vi "Auto Loop 1.vi"(2 "Auto State":u8, 3 "Call Context":T4) -> (0 "Loop 1 Data":T1, 1 "SubState 1":T2)   [LabVIEW 2014]
uses:
  <vilib>/Rock Robotics/WPI/DriverStation/WPI_DriverStationDerivedRobotMode.ctl
  typedefs/state machine/subStates.ctl
  typedefs/loop datatypes/Loop 1 Datatype.ctl
  typedefs/lift/lift command.ctl
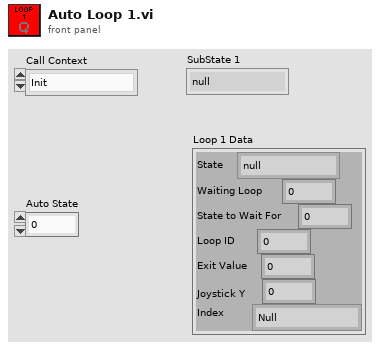
[diagram p1: front panel]
types:
  T1 = typedef "Loop 1 Datatype.ctl" = cluster{"State":T2, "Waiting Loop":i32, "State to Wait For":i32, "Loop ID":i32, "Exit Value":i32, "Joystick Y":dbl, "Index":T3}
  T2 = typedef "subStates.ctl" = enum16{"null", "wait", "driver control", "auto", "manual override", "hold position", "rotate", "test", "end"}
  T3 = typedef "lift command.ctl" = enum16{"Null", "Index Up", "Index Down", "Go To Home", "Cap 4 Stack", "Container Index Up", "Container Index Down", "Autonomous"}
  T4 = typedef "WPI_DriverStationDerivedRobotMode.ctl" = enum16{"Init", "Execute", "Stop"}
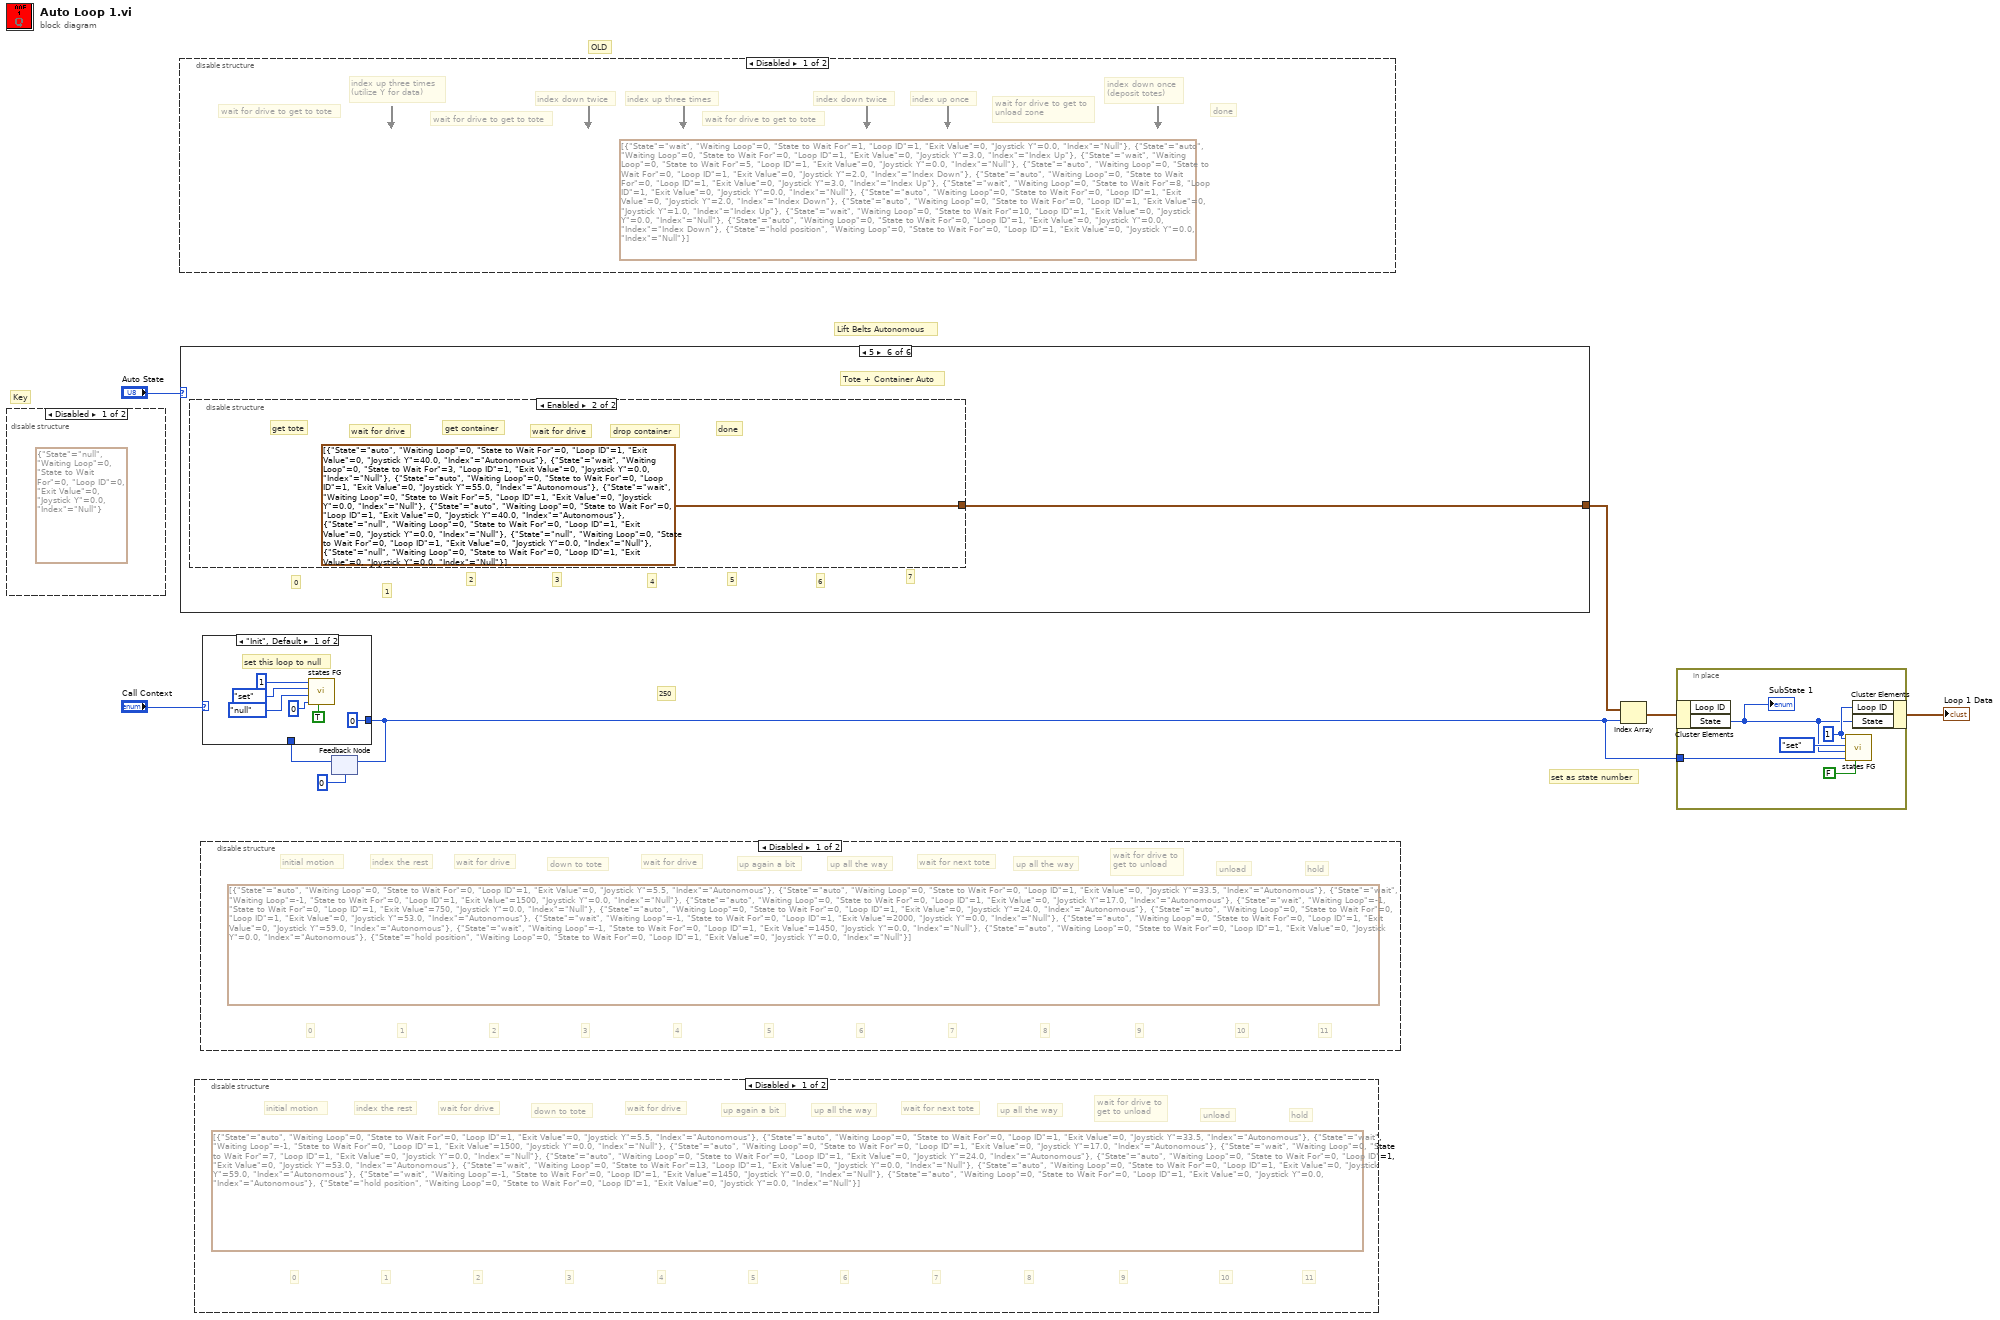
[diagram p0: block diagram]
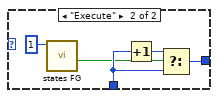
[diagram p6: hidden frame]
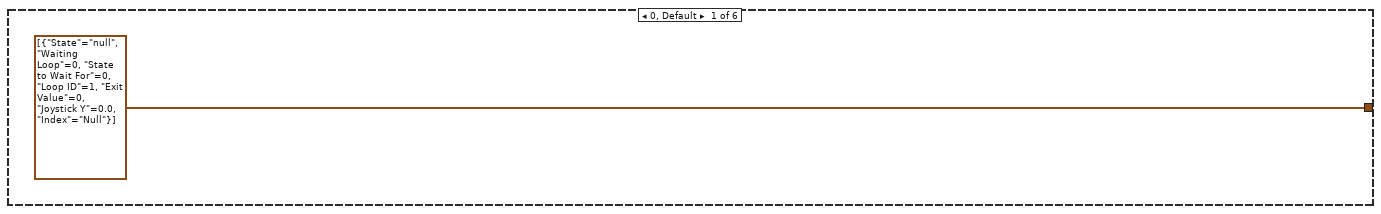
[diagram p7: hidden frame]
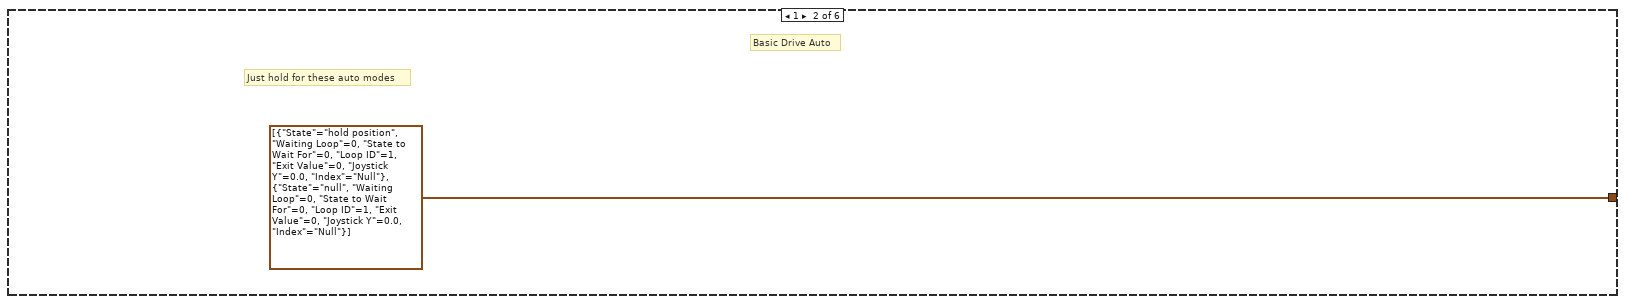
[diagram p8: hidden frame]
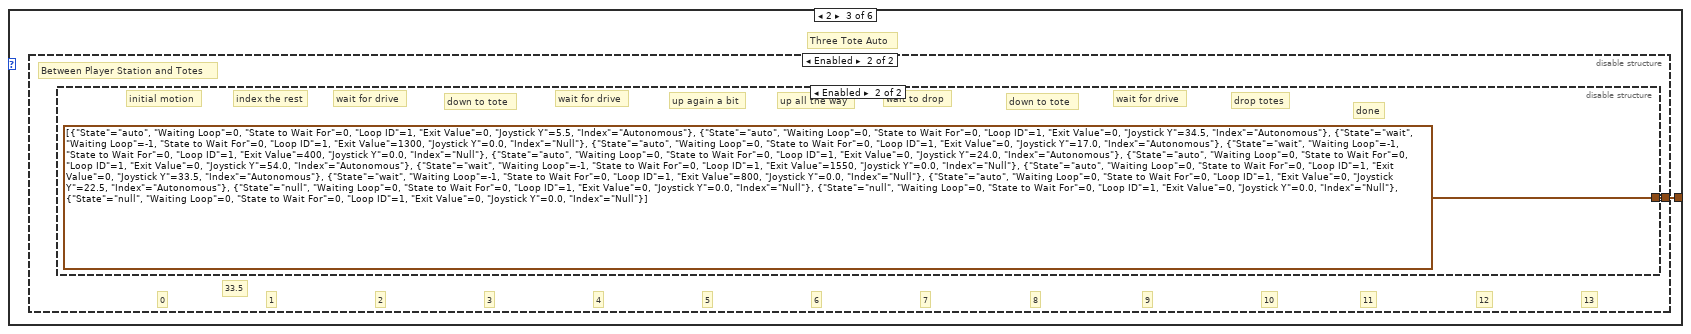
[diagram p9: hidden frame]
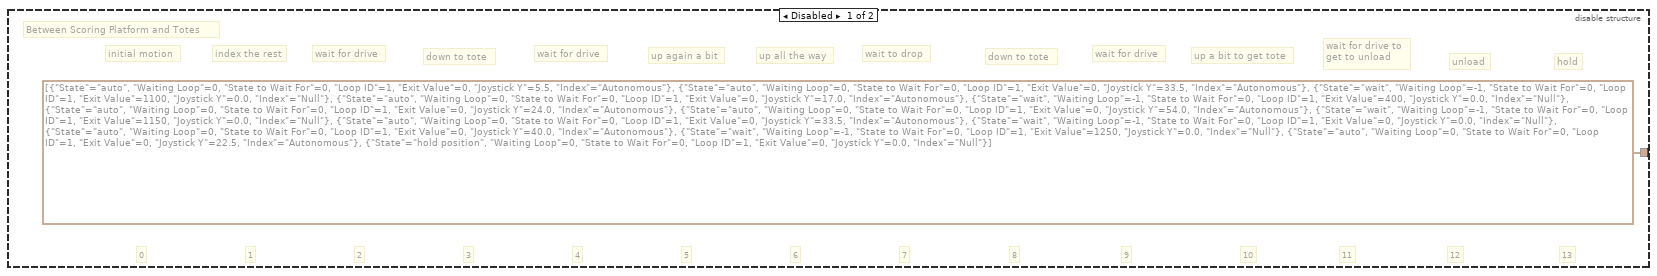
[diagram p10: hidden frame]
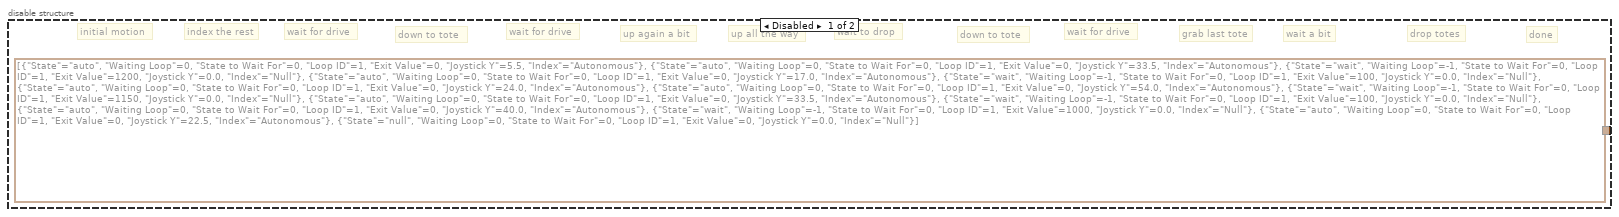
[diagram p11: hidden frame]
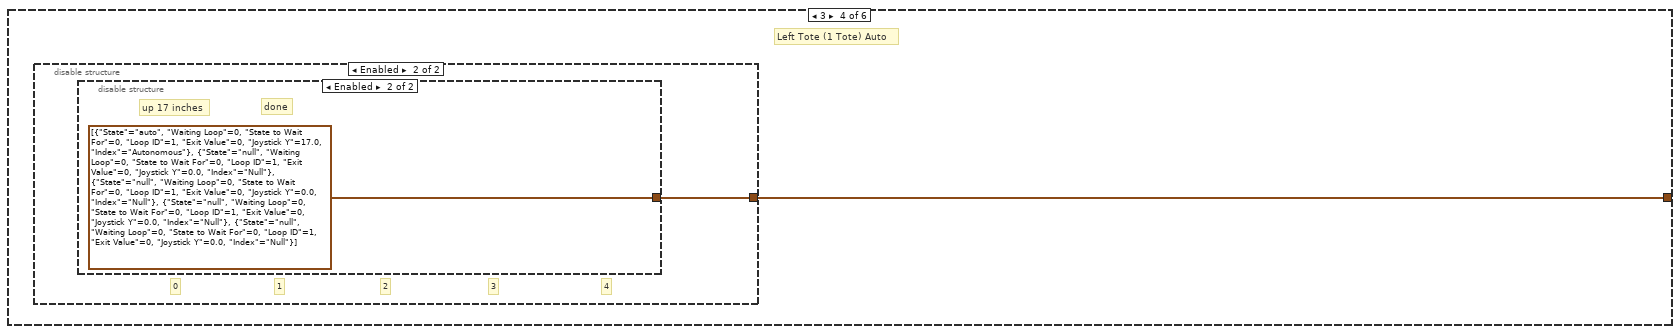
[diagram p12: hidden frame]
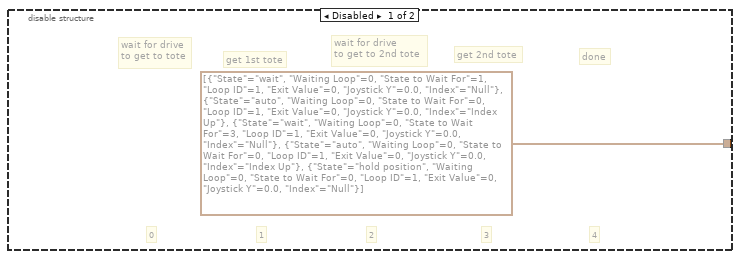
[diagram p13: hidden frame]
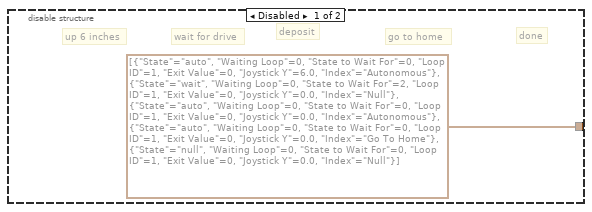
[diagram p14: hidden frame]
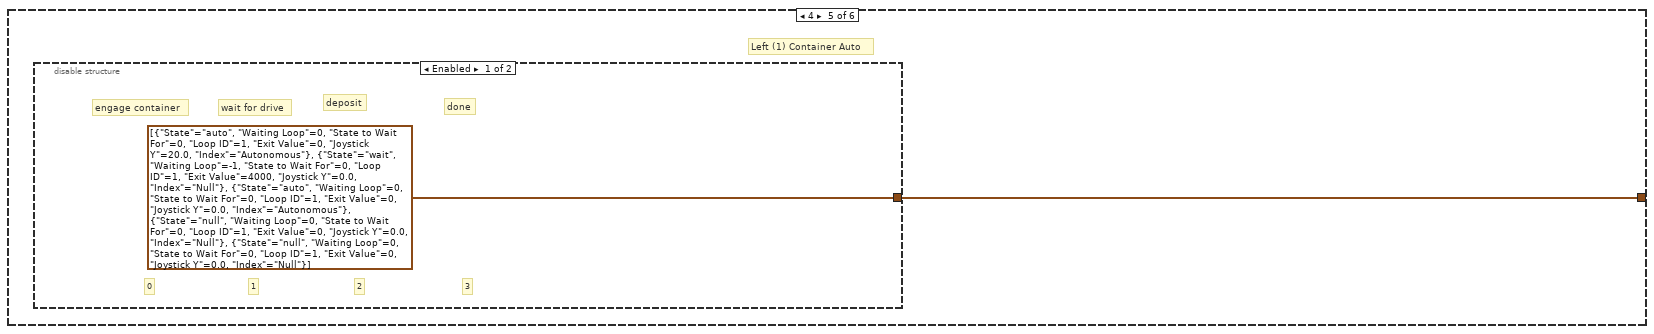
[diagram p15: hidden frame]
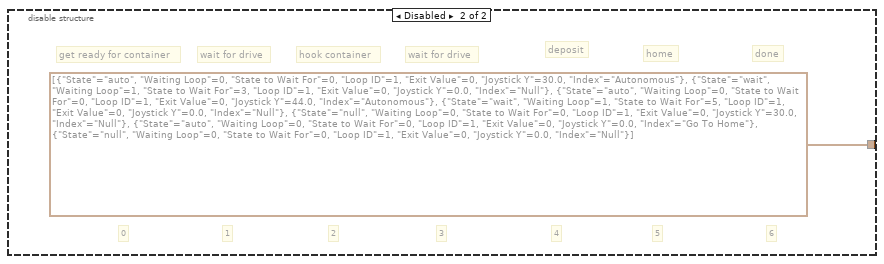
[diagram p16: hidden frame]
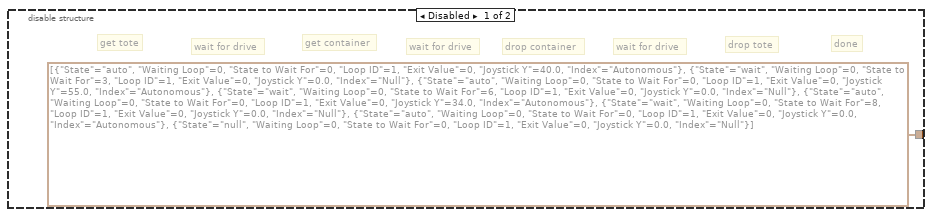
[diagram p17: hidden frame]
diagram:
  # "250"
  # "OLD"
  # "set as state number"
  # "Key"
  # "Lift Belts Autonomous"
  n1 = disable-structure shown="Disabled" {
    frame Disabled {
      (unwired) T1 {"State"=enum."null", "Waiting Loop"=0, "State to Wait For"=0, "Loop ID"=0, "Exit Value"=0, "Joystick Y"=0.0, "Index"=enum."Null"} ("Loop 1 Data")
    }
    frame Enabled {
    }
  }
  n2 = disable-structure shown="Disabled" {
    frame Disabled {
      (unwired) T1[] [{"State"=enum."wait", "Waiting Loop"=0, "State to Wait For"=1, "Loop ID"=1, "Exit Value"=0, "Joystick Y"=0.0, "Index"=enum."Null"}, {"State"=enum."auto", "Waiting Loop"=0, "State to Wait For"=0, "Loop ID"=1, "Exit Value"=0, "Joystick Y"=3.0, "Index"=enum."Index Up"}, {"State"=enum."wait", "Waiting Loop"=0, "State to Wait For"=5, "Loop ID"=1, "Exit Value"=0, "Joystick Y"=0.0, "Index"=enum."Null"}, {"State"=enum."auto", "Waiting Loop"=0, "State to Wait For"=0, "Loop ID"=1, "Exit Value"=0, "Joystick Y"=2.0, "Index"=enum."Index Down"}, {"State"=enum."auto", "Waiting Loop"=0, "State to Wait For"=0, "Loop ID"=1, "Exit Value"=0, "Joystick Y"=3.0, "Index"=enum."Index Up"}, {"State"=enum."wait", "Waiting Loop"=0, "State to Wait For"=8, "Loop ID"=1, "Exit Value"=0, "Joystick Y"=0.0, "Index"=enum."Null"}, {"State"=enum."auto", "Waiting Loop"=0, "State to Wait For"=0, "Loop ID"=1, "Exit Value"=0, "Joystick Y"=2.0, "Index"=enum."Index Down"}, {"State"=enum."auto", "Waiting Loop"=0, "State to Wait For"=0, "Loop ID"=1, "Exit Value"=0, "Joystick Y"=1.0, "Index"=enum."Index Up"}, {"State"=enum."wait", "Waiting Loop"=0, "State to Wait For"=10, "Loop ID"=1, "Exit Value"=0, "Joystick Y"=0.0, "Index"=enum."Null"}, {"State"=enum."auto", "Waiting Loop"=0, "State to Wait For"=0, "Loop ID"=1, "Exit Value"=0, "Joystick Y"=0.0, "Index"=enum."Index Down"}, {"State"=enum."hold position", "Waiting Loop"=0, "State to Wait For"=0, "Loop ID"=1, "Exit Value"=0, "Joystick Y"=0.0, "Index"=enum."Null"}]
      # "done"
      # "index down once\n(deposit totes)"
      # "wait for drive to get to\nunload zone"
      # "index up once"
      # "index down twice"
      # "wait for drive to get to tote"
      # "index up three times"
      # "index down twice"
      # "wait for drive to get to tote"
      # "index up three times \n(utilize Y for data)"
      # "wait for drive to get to tote"
    }
    frame Enabled {
    }
  }
  n3 = case shown="5" "Auto State" {
    tunnel: [T1[] [{"State"=enum."null", "Waiting Loop"=0, "State to Wait For"=0, "Loop ID"=1, "Exit Value"=0, "Joystick Y"=0.0, "Index"=enum."Null"}] T1[] [{"State"=enum."hold position", "Waiting Loop"=0, "State to Wait For"=0, "Loop ID"=1, "Exit Value"=0, "Joystick Y"=0.0, "Index"=enum."Null"}, {"State"=enum."null", "Waiting Loop"=0, "State to Wait For"=0, "Loop ID"=1, "Exit Value"=0, "Joystick Y"=0.0, "Index"=enum."Null"}] w11 w16 w21 w24] -> w4
    frame 0, Default {
    }
    frame 1 {
      # "Basic Drive Auto"
      # "Just hold for these auto modes"
    }
    frame 2 {
      # "Three Tote Auto"
      n4 = disable-structure shown="Enabled" {
        disable-tunnel: [T1[] [{"State"=enum."auto", "Waiting Loop"=0, "State to Wait For"=0, "Loop ID"=1, "Exit Value"=0, "Joystick Y"=5.5, "Index"=enum."Autonomous"}, {"State"=enum."auto", "Waiting Loop"=0, "State to Wait For"=0, "Loop ID"=1, "Exit Value"=0, "Joystick Y"=33.5, "Index"=enum."Autonomous"}, {"State"=enum."wait", "Waiting Loop"=-1, "State to Wait For"=0, "Loop ID"=1, "Exit Value"=1100, "Joystick Y"=0.0, "Index"=enum."Null"}, {"State"=enum."auto", "Waiting Loop"=0, "State to Wait For"=0, "Loop ID"=1, "Exit Value"=0, "Joystick Y"=17.0, "Index"=enum."Autonomous"}, {"State"=enum."wait", "Waiting Loop"=-1, "State to Wait For"=0, "Loop ID"=1, "Exit Value"=400, "Joystick Y"=0.0, "Index"=enum."Null"}, {"State"=enum."auto", "Waiting Loop"=0, "State to Wait For"=0, "Loop ID"=1, "Exit Value"=0, "Joystick Y"=24.0, "Index"=enum."Autonomous"}, {"State"=enum."auto", "Waiting Loop"=0, "State to Wait For"=0, "Loop ID"=1, "Exit Value"=0, "Joystick Y"=54.0, "Index"=enum."Autonomous"}, {"State"=enum."wait", "Waiting Loop"=-1, "State to Wait For"=0, "Loop ID"=1, "Exit Value"=1150, "Joystick Y"=0.0, "Index"=enum."Null"}, {"State"=enum."auto", "Waiting Loop"=0, "State to Wait For"=0, "Loop ID"=1, "Exit Value"=0, "Joystick Y"=33.5, "Index"=enum."Autonomous"}, {"State"=enum."wait", "Waiting Loop"=-1, "State to Wait For"=0, "Loop ID"=1, "Exit Value"=0, "Joystick Y"=0.0, "Index"=enum."Null"}, {"State"=enum."auto", "Waiting Loop"=0, "State to Wait For"=0, "Loop ID"=1, "Exit Value"=0, "Joystick Y"=40.0, "Index"=enum."Autonomous"}, {"State"=enum."wait", "Waiting Loop"=-1, "State to Wait For"=0, "Loop ID"=1, "Exit Value"=1250, "Joystick Y"=0.0, "Index"=enum."Null"}, {"State"=enum."auto", "Waiting Loop"=0, "State to Wait For"=0, "Loop ID"=1, "Exit Value"=0, "Joystick Y"=22.5, "Index"=enum."Autonomous"}, {"State"=enum."hold position", "Waiting Loop"=0, "State to Wait For"=0, "Loop ID"=1, "Exit Value"=0, "Joystick Y"=0.0, "Index"=enum."Null"}] w13] -> w11
        frame Disabled {
          # "Between Scoring Platform and Totes"
          # "13"
          # "12"
          # "wait for drive"
          # "down to tote"
          # "11"
          # "hold"
          # "10"
          # "9"
          # "8"
          # "wait for drive to\nget to unload"
          # "up a bit to get tote"
          # "wait to drop"
          # "unload"
          # "wait for drive"
          # "up all the way"
          # "up again a bit"
          # "down to tote"
          # "wait for drive"
          # "index the rest"
          # "initial motion"
          # "7"
          # "6"
          # "5"
          # "4"
          # "3"
          # "2"
          # "1"
          # "0"
        }
        frame Enabled {
          # "33.5"
          # "13"
          # "12"
          # "Between Player Station and Totes"
          # "11"
          # "10"
          # "9"
          # "8"
          # "7"
          # "6"
          # "5"
          # "4"
          # "3"
          # "2"
          # "1"
          # "0"
          n5 = disable-structure shown="Enabled" {
            disable-tunnel: [T1[] [{"State"=enum."auto", "Waiting Loop"=0, "State to Wait For"=0, "Loop ID"=1, "Exit Value"=0, "Joystick Y"=5.5, "Index"=enum."Autonomous"}, {"State"=enum."auto", "Waiting Loop"=0, "State to Wait For"=0, "Loop ID"=1, "Exit Value"=0, "Joystick Y"=33.5, "Index"=enum."Autonomous"}, {"State"=enum."wait", "Waiting Loop"=-1, "State to Wait For"=0, "Loop ID"=1, "Exit Value"=1200, "Joystick Y"=0.0, "Index"=enum."Null"}, {"State"=enum."auto", "Waiting Loop"=0, "State to Wait For"=0, "Loop ID"=1, "Exit Value"=0, "Joystick Y"=17.0, "Index"=enum."Autonomous"}, {"State"=enum."wait", "Waiting Loop"=-1, "State to Wait For"=0, "Loop ID"=1, "Exit Value"=100, "Joystick Y"=0.0, "Index"=enum."Null"}, {"State"=enum."auto", "Waiting Loop"=0, "State to Wait For"=0, "Loop ID"=1, "Exit Value"=0, "Joystick Y"=24.0, "Index"=enum."Autonomous"}, {"State"=enum."auto", "Waiting Loop"=0, "State to Wait For"=0, "Loop ID"=1, "Exit Value"=0, "Joystick Y"=54.0, "Index"=enum."Autonomous"}, {"State"=enum."wait", "Waiting Loop"=-1, "State to Wait For"=0, "Loop ID"=1, "Exit Value"=1150, "Joystick Y"=0.0, "Index"=enum."Null"}, {"State"=enum."auto", "Waiting Loop"=0, "State to Wait For"=0, "Loop ID"=1, "Exit Value"=0, "Joystick Y"=33.5, "Index"=enum."Autonomous"}, {"State"=enum."wait", "Waiting Loop"=-1, "State to Wait For"=0, "Loop ID"=1, "Exit Value"=100, "Joystick Y"=0.0, "Index"=enum."Null"}, {"State"=enum."auto", "Waiting Loop"=0, "State to Wait For"=0, "Loop ID"=1, "Exit Value"=0, "Joystick Y"=40.0, "Index"=enum."Autonomous"}, {"State"=enum."wait", "Waiting Loop"=-1, "State to Wait For"=0, "Loop ID"=1, "Exit Value"=1000, "Joystick Y"=0.0, "Index"=enum."Null"}, {"State"=enum."auto", "Waiting Loop"=0, "State to Wait For"=0, "Loop ID"=1, "Exit Value"=0, "Joystick Y"=22.5, "Index"=enum."Autonomous"}, {"State"=enum."null", "Waiting Loop"=0, "State to Wait For"=0, "Loop ID"=1, "Exit Value"=0, "Joystick Y"=0.0, "Index"=enum."Null"}] T1[] [{"State"=enum."auto", "Waiting Loop"=0, "State to Wait For"=0, "Loop ID"=1, "Exit Value"=0, "Joystick Y"=5.5, "Index"=enum."Autonomous"}, {"State"=enum."auto", "Waiting Loop"=0, "State to Wait For"=0, "Loop ID"=1, "Exit Value"=0, "Joystick Y"=34.5, "Index"=enum."Autonomous"}, {"State"=enum."wait", "Waiting Loop"=-1, "State to Wait For"=0, "Loop ID"=1, "Exit Value"=1300, "Joystick Y"=0.0, "Index"=enum."Null"}, {"State"=enum."auto", "Waiting Loop"=0, "State to Wait For"=0, "Loop ID"=1, "Exit Value"=0, "Joystick Y"=17.0, "Index"=enum."Autonomous"}, {"State"=enum."wait", "Waiting Loop"=-1, "State to Wait For"=0, "Loop ID"=1, "Exit Value"=400, "Joystick Y"=0.0, "Index"=enum."Null"}, {"State"=enum."auto", "Waiting Loop"=0, "State to Wait For"=0, "Loop ID"=1, "Exit Value"=0, "Joystick Y"=24.0, "Index"=enum."Autonomous"}, {"State"=enum."auto", "Waiting Loop"=0, "State to Wait For"=0, "Loop ID"=1, "Exit Value"=0, "Joystick Y"=54.0, "Index"=enum."Autonomous"}, {"State"=enum."wait", "Waiting Loop"=-1, "State to Wait For"=0, "Loop ID"=1, "Exit Value"=1550, "Joystick Y"=0.0, "Index"=enum."Null"}, {"State"=enum."auto", "Waiting Loop"=0, "State to Wait For"=0, "Loop ID"=1, "Exit Value"=0, "Joystick Y"=33.5, "Index"=enum."Autonomous"}, {"State"=enum."wait", "Waiting Loop"=-1, "State to Wait For"=0, "Loop ID"=1, "Exit Value"=800, "Joystick Y"=0.0, "Index"=enum."Null"}, {"State"=enum."auto", "Waiting Loop"=0, "State to Wait For"=0, "Loop ID"=1, "Exit Value"=0, "Joystick Y"=22.5, "Index"=enum."Autonomous"}, {"State"=enum."null", "Waiting Loop"=0, "State to Wait For"=0, "Loop ID"=1, "Exit Value"=0, "Joystick Y"=0.0, "Index"=enum."Null"}, {"State"=enum."null", "Waiting Loop"=0, "State to Wait For"=0, "Loop ID"=1, "Exit Value"=0, "Joystick Y"=0.0, "Index"=enum."Null"}, {"State"=enum."null", "Waiting Loop"=0, "State to Wait For"=0, "Loop ID"=1, "Exit Value"=0, "Joystick Y"=0.0, "Index"=enum."Null"}]] -> w13
            frame Disabled {
              # "drop totes"
              # "wait a bit"
              # "wait for drive"
              # "down to tote"
              # "done"
              # "grab last tote"
              # "wait to drop"
              # "wait for drive"
              # "up all the way"
              # "up again a bit"
              # "down to tote"
              # "wait for drive"
              # "index the rest"
              # "initial motion"
            }
            frame Enabled {
              # "done"
              # "drop totes"
              # "wait for drive"
              # "down to tote"
              # "wait to drop"
              # "wait for drive"
              # "up all the way"
              # "up again a bit"
              # "down to tote"
              # "wait for drive"
              # "index the rest"
              # "initial motion"
            }
          }
        }
      }
    }
    frame 3 {
      # "Left Tote (1 Tote) Auto"
      n6 = disable-structure shown="Enabled" {
        disable-tunnel: [T1[] [{"State"=enum."wait", "Waiting Loop"=0, "State to Wait For"=1, "Loop ID"=1, "Exit Value"=0, "Joystick Y"=0.0, "Index"=enum."Null"}, {"State"=enum."auto", "Waiting Loop"=0, "State to Wait For"=0, "Loop ID"=1, "Exit Value"=0, "Joystick Y"=0.0, "Index"=enum."Index Up"}, {"State"=enum."wait", "Waiting Loop"=0, "State to Wait For"=3, "Loop ID"=1, "Exit Value"=0, "Joystick Y"=0.0, "Index"=enum."Null"}, {"State"=enum."auto", "Waiting Loop"=0, "State to Wait For"=0, "Loop ID"=1, "Exit Value"=0, "Joystick Y"=0.0, "Index"=enum."Index Up"}, {"State"=enum."hold position", "Waiting Loop"=0, "State to Wait For"=0, "Loop ID"=1, "Exit Value"=0, "Joystick Y"=0.0, "Index"=enum."Null"}] w18] -> w16
        frame Disabled {
          # "done"
          # "4"
          # "3"
          # "get 2nd tote"
          # "wait for drive\nto get to 2nd tote"
          # "get 1st tote"
          # "wait for drive\nto get to tote"
          # "2"
          # "1"
          # "0"
        }
        frame Enabled {
          # "4"
          # "3"
          # "2"
          # "1"
          # "0"
          n7 = disable-structure shown="Enabled" {
            disable-tunnel: [T1[] [{"State"=enum."auto", "Waiting Loop"=0, "State to Wait For"=0, "Loop ID"=1, "Exit Value"=0, "Joystick Y"=6.0, "Index"=enum."Autonomous"}, {"State"=enum."wait", "Waiting Loop"=0, "State to Wait For"=2, "Loop ID"=1, "Exit Value"=0, "Joystick Y"=0.0, "Index"=enum."Null"}, {"State"=enum."auto", "Waiting Loop"=0, "State to Wait For"=0, "Loop ID"=1, "Exit Value"=0, "Joystick Y"=0.0, "Index"=enum."Autonomous"}, {"State"=enum."auto", "Waiting Loop"=0, "State to Wait For"=0, "Loop ID"=1, "Exit Value"=0, "Joystick Y"=0.0, "Index"=enum."Go To Home"}, {"State"=enum."null", "Waiting Loop"=0, "State to Wait For"=0, "Loop ID"=1, "Exit Value"=0, "Joystick Y"=0.0, "Index"=enum."Null"}] T1[] [{"State"=enum."auto", "Waiting Loop"=0, "State to Wait For"=0, "Loop ID"=1, "Exit Value"=0, "Joystick Y"=17.0, "Index"=enum."Autonomous"}, {"State"=enum."null", "Waiting Loop"=0, "State to Wait For"=0, "Loop ID"=1, "Exit Value"=0, "Joystick Y"=0.0, "Index"=enum."Null"}, {"State"=enum."null", "Waiting Loop"=0, "State to Wait For"=0, "Loop ID"=1, "Exit Value"=0, "Joystick Y"=0.0, "Index"=enum."Null"}, {"State"=enum."null", "Waiting Loop"=0, "State to Wait For"=0, "Loop ID"=1, "Exit Value"=0, "Joystick Y"=0.0, "Index"=enum."Null"}, {"State"=enum."null", "Waiting Loop"=0, "State to Wait For"=0, "Loop ID"=1, "Exit Value"=0, "Joystick Y"=0.0, "Index"=enum."Null"}]] -> w18
            frame Disabled {
              # "go to home"
              # "done"
              # "deposit"
              # "wait for drive"
              # "up 6 inches"
            }
            frame Enabled {
              # "6"
              # "done"
              # "up 17 inches"
            }
          }
        }
      }
    }
    frame 4 {
      # "Left (1) Container Auto"
      n8 = disable-structure shown="Enabled" {
        disable-tunnel: [T1[] [{"State"=enum."auto", "Waiting Loop"=0, "State to Wait For"=0, "Loop ID"=1, "Exit Value"=0, "Joystick Y"=20.0, "Index"=enum."Autonomous"}, {"State"=enum."wait", "Waiting Loop"=-1, "State to Wait For"=0, "Loop ID"=1, "Exit Value"=4000, "Joystick Y"=0.0, "Index"=enum."Null"}, {"State"=enum."auto", "Waiting Loop"=0, "State to Wait For"=0, "Loop ID"=1, "Exit Value"=0, "Joystick Y"=0.0, "Index"=enum."Autonomous"}, {"State"=enum."null", "Waiting Loop"=0, "State to Wait For"=0, "Loop ID"=1, "Exit Value"=0, "Joystick Y"=0.0, "Index"=enum."Null"}, {"State"=enum."null", "Waiting Loop"=0, "State to Wait For"=0, "Loop ID"=1, "Exit Value"=0, "Joystick Y"=0.0, "Index"=enum."Null"}] T1[] [{"State"=enum."auto", "Waiting Loop"=0, "State to Wait For"=0, "Loop ID"=1, "Exit Value"=0, "Joystick Y"=30.0, "Index"=enum."Autonomous"}, {"State"=enum."wait", "Waiting Loop"=1, "State to Wait For"=3, "Loop ID"=1, "Exit Value"=0, "Joystick Y"=0.0, "Index"=enum."Null"}, {"State"=enum."auto", "Waiting Loop"=0, "State to Wait For"=0, "Loop ID"=1, "Exit Value"=0, "Joystick Y"=44.0, "Index"=enum."Autonomous"}, {"State"=enum."wait", "Waiting Loop"=1, "State to Wait For"=5, "Loop ID"=1, "Exit Value"=0, "Joystick Y"=0.0, "Index"=enum."Null"}, {"State"=enum."null", "Waiting Loop"=0, "State to Wait For"=0, "Loop ID"=1, "Exit Value"=0, "Joystick Y"=30.0, "Index"=enum."Null"}, {"State"=enum."auto", "Waiting Loop"=0, "State to Wait For"=0, "Loop ID"=1, "Exit Value"=0, "Joystick Y"=0.0, "Index"=enum."Go To Home"}, {"State"=enum."null", "Waiting Loop"=0, "State to Wait For"=0, "Loop ID"=1, "Exit Value"=0, "Joystick Y"=0.0, "Index"=enum."Null"}]] -> w21
        frame Enabled {
          # "3"
          # "done"
          # "2"
          # "deposit"
          # "1"
          # "wait for drive"
          # "engage container"
          # "0"
        }
        frame Disabled {
          # "6"
          # "home"
          # "5"
          # "4"
          # "wait for drive"
          # "wait for drive"
          # "3"
          # "done"
          # "2"
          # "deposit"
          # "1"
          # "hook container"
          # "get ready for container"
          # "0"
        }
      }
    }
    frame 5 {
      # "7"
      # "6"
      # "5"
      # "4"
      # "3"
      # "2"
      # "1"
      # "0"
      # "Tote + Container Auto"
      n9 = disable-structure shown="Enabled" {
        disable-tunnel: [T1[] [{"State"=enum."auto", "Waiting Loop"=0, "State to Wait For"=0, "Loop ID"=1, "Exit Value"=0, "Joystick Y"=40.0, "Index"=enum."Autonomous"}, {"State"=enum."wait", "Waiting Loop"=0, "State to Wait For"=3, "Loop ID"=1, "Exit Value"=0, "Joystick Y"=0.0, "Index"=enum."Null"}, {"State"=enum."auto", "Waiting Loop"=0, "State to Wait For"=0, "Loop ID"=1, "Exit Value"=0, "Joystick Y"=55.0, "Index"=enum."Autonomous"}, {"State"=enum."wait", "Waiting Loop"=0, "State to Wait For"=6, "Loop ID"=1, "Exit Value"=0, "Joystick Y"=0.0, "Index"=enum."Null"}, {"State"=enum."auto", "Waiting Loop"=0, "State to Wait For"=0, "Loop ID"=1, "Exit Value"=0, "Joystick Y"=34.0, "Index"=enum."Autonomous"}, {"State"=enum."wait", "Waiting Loop"=0, "State to Wait For"=8, "Loop ID"=1, "Exit Value"=0, "Joystick Y"=0.0, "Index"=enum."Null"}, {"State"=enum."auto", "Waiting Loop"=0, "State to Wait For"=0, "Loop ID"=1, "Exit Value"=0, "Joystick Y"=0.0, "Index"=enum."Autonomous"}, {"State"=enum."null", "Waiting Loop"=0, "State to Wait For"=0, "Loop ID"=1, "Exit Value"=0, "Joystick Y"=0.0, "Index"=enum."Null"}] T1[] [{"State"=enum."auto", "Waiting Loop"=0, "State to Wait For"=0, "Loop ID"=1, "Exit Value"=0, "Joystick Y"=40.0, "Index"=enum."Autonomous"}, {"State"=enum."wait", "Waiting Loop"=0, "State to Wait For"=3, "Loop ID"=1, "Exit Value"=0, "Joystick Y"=0.0, "Index"=enum."Null"}, {"State"=enum."auto", "Waiting Loop"=0, "State to Wait For"=0, "Loop ID"=1, "Exit Value"=0, "Joystick Y"=55.0, "Index"=enum."Autonomous"}, {"State"=enum."wait", "Waiting Loop"=0, "State to Wait For"=5, "Loop ID"=1, "Exit Value"=0, "Joystick Y"=0.0, "Index"=enum."Null"}, {"State"=enum."auto", "Waiting Loop"=0, "State to Wait For"=0, "Loop ID"=1, "Exit Value"=0, "Joystick Y"=40.0, "Index"=enum."Autonomous"}, {"State"=enum."null", "Waiting Loop"=0, "State to Wait For"=0, "Loop ID"=1, "Exit Value"=0, "Joystick Y"=0.0, "Index"=enum."Null"}, {"State"=enum."null", "Waiting Loop"=0, "State to Wait For"=0, "Loop ID"=1, "Exit Value"=0, "Joystick Y"=0.0, "Index"=enum."Null"}, {"State"=enum."null", "Waiting Loop"=0, "State to Wait For"=0, "Loop ID"=1, "Exit Value"=0, "Joystick Y"=0.0, "Index"=enum."Null"}]] -> w24
        frame Disabled {
          # "done"
          # "drop tote"
          # "wait for drive"
          # "drop container"
          # "wait for drive"
          # "get container"
          # "wait for drive"
          # "get tote"
        }
        frame Enabled {
          # "done"
          # "drop container"
          # "wait for drive"
          # "get container"
          # "wait for drive"
          # "get tote"
        }
      }
    }
  }
  n10 = disable-structure shown="Disabled" {
    frame Disabled {
      (unwired) T1[] [{"State"=enum."auto", "Waiting Loop"=0, "State to Wait For"=0, "Loop ID"=1, "Exit Value"=0, "Joystick Y"=5.5, "Index"=enum."Autonomous"}, {"State"=enum."auto", "Waiting Loop"=0, "State to Wait For"=0, "Loop ID"=1, "Exit Value"=0, "Joystick Y"=33.5, "Index"=enum."Autonomous"}, {"State"=enum."wait", "Waiting Loop"=-1, "State to Wait For"=0, "Loop ID"=1, "Exit Value"=1500, "Joystick Y"=0.0, "Index"=enum."Null"}, {"State"=enum."auto", "Waiting Loop"=0, "State to Wait For"=0, "Loop ID"=1, "Exit Value"=0, "Joystick Y"=17.0, "Index"=enum."Autonomous"}, {"State"=enum."wait", "Waiting Loop"=0, "State to Wait For"=7, "Loop ID"=1, "Exit Value"=0, "Joystick Y"=0.0, "Index"=enum."Null"}, {"State"=enum."auto", "Waiting Loop"=0, "State to Wait For"=0, "Loop ID"=1, "Exit Value"=0, "Joystick Y"=24.0, "Index"=enum."Autonomous"}, {"State"=enum."auto", "Waiting Loop"=0, "State to Wait For"=0, "Loop ID"=1, "Exit Value"=0, "Joystick Y"=53.0, "Index"=enum."Autonomous"}, {"State"=enum."wait", "Waiting Loop"=0, "State to Wait For"=13, "Loop ID"=1, "Exit Value"=0, "Joystick Y"=0.0, "Index"=enum."Null"}, {"State"=enum."auto", "Waiting Loop"=0, "State to Wait For"=0, "Loop ID"=1, "Exit Value"=0, "Joystick Y"=59.0, "Index"=enum."Autonomous"}, {"State"=enum."wait", "Waiting Loop"=-1, "State to Wait For"=0, "Loop ID"=1, "Exit Value"=1450, "Joystick Y"=0.0, "Index"=enum."Null"}, {"State"=enum."auto", "Waiting Loop"=0, "State to Wait For"=0, "Loop ID"=1, "Exit Value"=0, "Joystick Y"=0.0, "Index"=enum."Autonomous"}, {"State"=enum."hold position", "Waiting Loop"=0, "State to Wait For"=0, "Loop ID"=1, "Exit Value"=0, "Joystick Y"=0.0, "Index"=enum."Null"}]
      # "11"
      # "hold"
      # "10"
      # "9"
      # "8"
      # "wait for drive to\nget to unload"
      # "up all the way"
      # "wait for next tote"
      # "unload"
      # "wait for drive"
      # "up all the way"
      # "up again a bit"
      # "down to tote"
      # "wait for drive"
      # "index the rest"
      # "initial motion"
      # "7"
      # "6"
      # "5"
      # "4"
      # "3"
      # "2"
      # "1"
      # "0"
    }
    frame Enabled {
    }
  }
  n11 = disable-structure shown="Disabled" {
    frame Disabled {
      (unwired) T1[] [{"State"=enum."auto", "Waiting Loop"=0, "State to Wait For"=0, "Loop ID"=1, "Exit Value"=0, "Joystick Y"=5.5, "Index"=enum."Autonomous"}, {"State"=enum."auto", "Waiting Loop"=0, "State to Wait For"=0, "Loop ID"=1, "Exit Value"=0, "Joystick Y"=33.5, "Index"=enum."Autonomous"}, {"State"=enum."wait", "Waiting Loop"=-1, "State to Wait For"=0, "Loop ID"=1, "Exit Value"=1500, "Joystick Y"=0.0, "Index"=enum."Null"}, {"State"=enum."auto", "Waiting Loop"=0, "State to Wait For"=0, "Loop ID"=1, "Exit Value"=0, "Joystick Y"=17.0, "Index"=enum."Autonomous"}, {"State"=enum."wait", "Waiting Loop"=-1, "State to Wait For"=0, "Loop ID"=1, "Exit Value"=750, "Joystick Y"=0.0, "Index"=enum."Null"}, {"State"=enum."auto", "Waiting Loop"=0, "State to Wait For"=0, "Loop ID"=1, "Exit Value"=0, "Joystick Y"=24.0, "Index"=enum."Autonomous"}, {"State"=enum."auto", "Waiting Loop"=0, "State to Wait For"=0, "Loop ID"=1, "Exit Value"=0, "Joystick Y"=53.0, "Index"=enum."Autonomous"}, {"State"=enum."wait", "Waiting Loop"=-1, "State to Wait For"=0, "Loop ID"=1, "Exit Value"=2000, "Joystick Y"=0.0, "Index"=enum."Null"}, {"State"=enum."auto", "Waiting Loop"=0, "State to Wait For"=0, "Loop ID"=1, "Exit Value"=0, "Joystick Y"=59.0, "Index"=enum."Autonomous"}, {"State"=enum."wait", "Waiting Loop"=-1, "State to Wait For"=0, "Loop ID"=1, "Exit Value"=1450, "Joystick Y"=0.0, "Index"=enum."Null"}, {"State"=enum."auto", "Waiting Loop"=0, "State to Wait For"=0, "Loop ID"=1, "Exit Value"=0, "Joystick Y"=0.0, "Index"=enum."Autonomous"}, {"State"=enum."hold position", "Waiting Loop"=0, "State to Wait For"=0, "Loop ID"=1, "Exit Value"=0, "Joystick Y"=0.0, "Index"=enum."Null"}]
      # "11"
      # "hold"
      # "10"
      # "9"
      # "8"
      # "wait for drive to\nget to unload"
      # "up all the way"
      # "wait for next tote"
      # "unload"
      # "wait for drive"
      # "up all the way"
      # "up again a bit"
      # "down to tote"
      # "wait for drive"
      # "index the rest"
      # "initial motion"
      # "7"
      # "6"
      # "5"
      # "4"
      # "3"
      # "2"
      # "1"
      # "0"
    }
    frame Enabled {
    }
  }
  n12 = feedback #1(0) -> (w8:i32)
  n13 = case shown="\"Init\", Default" "Call Context" {
    tunnel: w8 -> [_ w36]
    tunnel: [0 w34] -> w1
    frame "Init", Default {
      # "set this loop to null"
      n14 = call "states FG.vi"("exit in"=TRUE, "state # in"=0, "subState in"=subStates."null", "menu (get)"=enum16{"set", "get"}."set", "Loop ID"=1) -> ()  [unwired: 3 in, 4 out]
    }
    frame "Execute" {
      n15 = call "states FG.vi"("Loop ID"=1) -> ("exit out"=w33:bool)  [unwired: 7 in, 3 out]
      n16 = Increment(x=w36) -> (x+1=w35:i32)
      n17 = Select(t=w35, s=w33, f=w36) -> (s? t:f=w34:i32)
    }
  }
  n18 = feedback-in #1(w1) -> ()
  n19 = Index Array(array=w4, index=w1) -> (element=w3:T1)
  n20 = in-place {
    in-place-border: w1 -> [w38]
    w40 = 1 ("Loop ID")
    n21 = in-place-cluster #2(w3) -> ("State"=w39:T2)  [unwired: 1 out]
    "SubState 1" <- w39
    n22 = call "states FG.vi"("exit in"=FALSE, "state # in"=w38, "subState in"=w39, "menu (get)"=enum16{"set", "get"}."set", "Loop ID"=w40) -> ()  [unwired: 3 in, 4 out]
    n23 = in-place-cluster #2("Loop ID"=w40, "State"=w39) -> (→"Loop 1 Data":T1)
  }
